vi "Auto-Refresh Start.vi"(8 "error in (no error)":errorcluster, 11 "MSX-E3701 in":refnum<class "MSX-E3701.lvclass">) -> (0 "error out":errorcluster, 3 "MSX-E3701 out":refnum<class "MSX-E3701.lvclass">)   [LabVIEW 2014, in "MSX-E3701.lvlib" / "MSX-E3701.lvclass"]
doc: "Adquiere la información necesaria y se la envía al web server para configurar el modo de adquisición de datos."
uses:
  MSX-E3701.lvclass
  MSX-E3701.lvclass/MSX-E3701.ctl
  API/MSX-E3701_dll.lvlib
  DriverMasterSync/build/DriverMasterSync.lvlibp/Modules/HAL/DriverMasterSync/DriverMasterSyncClass/DriverMasterSync.lvclass
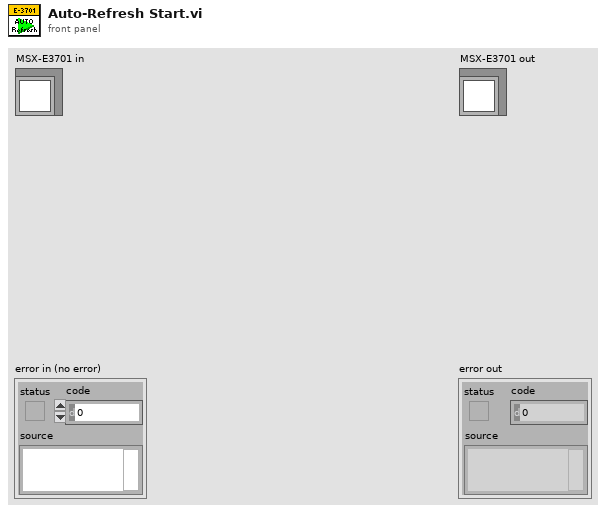
[diagram p1: front panel]
types:
  T1 = typedef "DriverMasterSync.lvlibp/HAL Config Data.ctl" = cluster{"HWSync Index":u32, "Driver Name":string, "Channel Mask":u64}
  T2 = typedef "MSX-E3701_dll.lvlib/Connection Data.ctl" = cluster{"MX370x refnum":refnum<k24>, "IP":string, "Connection ID ":refnum<k5>, "MXCommon refnum":refnum<k24>}
  T3 = typedef "MSX-E3701_dll.lvlib/Config Data.ctl" = cluster{"Auto Refresh":cluster{"Average Mode":u64, "Average Value":u64, "Division Factor":u64, "Trigger Action":u64, "Hardware Trigger Count":u64, "Hardware Trigger Filter Time":u64, "By Trigger Nbr Of Seq To Acquire":u64, "Time stamp":bool, "Analog Output(mm)":bool, "Invert value":bool}, "Gain":sgl[], "Offset":sgl[], "Index":u64, "Range":sgl, "Sequence":cluster{"Division Factor":u64, "Nbr Of Sequence":u64, "Nbr Max Sequence To Transfer":u64, "Sequence.Delay Mode":u64, "Delay Time Unit":u64, "Delay Value":u64, "Trigger Action":u64, "Hardware Trigger Count":u64, "Hardware Trigger Filter Time":u64, "By Trigger Nbr Of Seq To Acquire":u64, "Time stamp":bool, "Sequence counter information":bool, "Analog Output(mm)":bool, "Invert value":bool, "Relative Time Stamp":bool, "Hardware trigger information":bool}, "Enable DIO":bool}
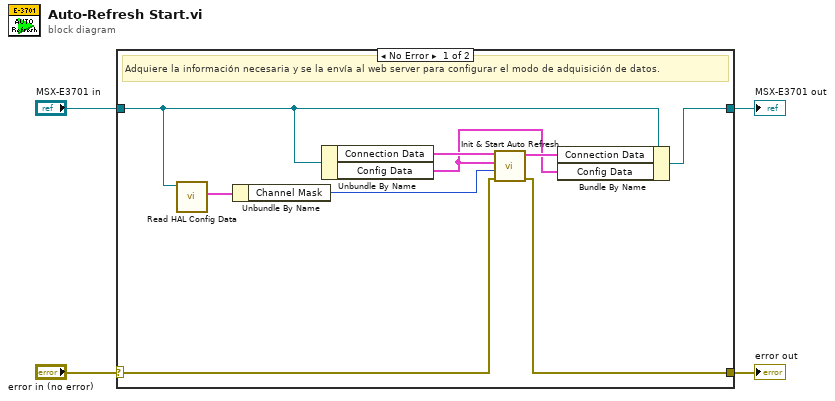
[diagram p0: block diagram]
diagram:
  n1 = case shown="No Error" "error in (no error)" {
    selector: "error in (no error)" -> [w10 w15]
    tunnel: [w9 w15] -> w3
    tunnel: [w12 w14] -> w1
    tunnel: "MSX-E3701 in" -> [w8 w14]
    frame No Error {
      # "Adquiere la información necesaria y se la envía al web server para configurar el modo de adquisición de datos."
      n2 = call "Read HAL Config Data.vi"("DriverMasterSync in"=w8) -> ("HAL Config Data"=w7:T1)  [unwired: 8 in, 2 out]
      n3 = Unbundle By Name(w7) -> ("Channel Mask"=w6:u64)
      n4 = Unbundle By Name(w8) -> ("Connection Data"=w13:T2, "Config Data"=w5:T3)
      n5 = call "Init & Start Auto Refresh.vi"("error in (no error)"=w10, "Channel Mask"=w6, "Config Data"=w5, "Connection Data In"=w13) -> ("error out"=w9:errorcluster, "Connection Data Out"=w11:T2)  [unwired: 6 in]
      n6 = Bundle By Name(cluster=w8, "Connection Data"=w11, "Config Data"=w5) -> (w12:refnum<class "MSX-E3701.lvclass">)
    }
    frame Error {
    }
  }
  "error out" <- w3
  "MSX-E3701 out" <- w1
